vi "Home one linear axis relative to limit.vi"(6 "Set Home limit":bool caption="Set Home relative to this limit", 8 "error in (no error)":errorcluster, 9 "Axis (1..4)":u16(ring)=1 items=["X"=1, "Y"=2, "Z"=3, "Rotary"=4], 10 "Absolute 0 position, counts":i32=-200 caption="Absolute 0 position from limit switch, counts", 11 "VISA resource name":refnum<visa-resource-name>) -> (0 "error out":errorcluster, 1 "current position, counts":i32, 3 "VISA resource out":refnum<visa-resource-name>)   [LabVIEW 2017]
panel:
  # "< always positive number here"
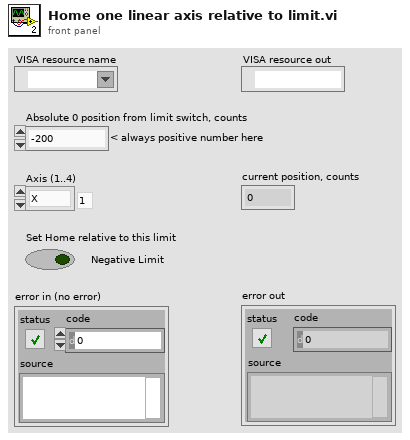
[diagram p1: front panel]
types:
  T1 = enum16{"Cmd-Response", "Write Only", "Read Only"}
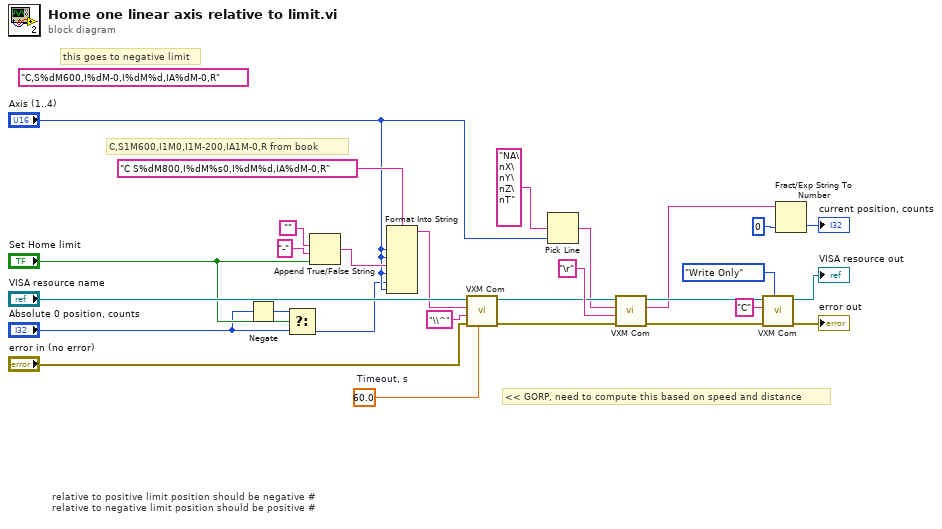
[diagram p0: block diagram]
diagram:
  (unwired) "C,S%dM600,I%dM-0,I%dM%d,IA%dM-0,R" ("Write Buffer")
  w11 = 60.0  # Timeout, s
  # "relative to positive limit position should be negative #\nrelative to negative limit position should be positive #"
  # "C,S1M600,I1M0,I1M-200,IA1M-0,R from book"
  # "this goes to negative limit"
  # "<< GORP, need to compute this based on speed and distance"
  n1 = Negate(x="Absolute 0 position, counts") -> (-x=w1:i32)
  n2 = Select(t=w1, s="Set Home limit", f="Absolute 0 position, counts") -> (s? t:f=w4:i32)
  n3 = Append True/False String(1:"Set Home limit", 2:"-" ("false string"), 3:"") -> (0:w6:string)  [unwired: 1 in]
  n4 = Format Into String(format string="C S%dM800,I%dM%s0,I%dM%d,IA%dM-0,R" ("Write Buffer"), "Axis (1..4)", "Axis (1..4)", w6, "Axis (1..4)", w4, "Axis (1..4)") -> (resulting string=w27:string)  [unwired: 2 in, 1 out]
  n5 = call "VXM Com.vi"("Timeout, s"=w11, "error in (no error)"="error in (no error)", "Termination String ('/' codes)"="\\^", "Write Buffer ('/' codes)"=w27, "VISA resource name"="VISA resource name") -> ("error out"=w19:errorcluster, "VISA resource out"=w23:refnum<visa-resource-name>)  [unwired: 4 in, 1 out]
  n6 = Pick Line(multi-line string="NA\nX\nY\nZ\nT", line index="Axis (1..4)") -> (output string=w13:string)  [unwired: 1 in]
  n7 = call "VXM Com.vi"("error in (no error)"=w19, "Termination String ('/' codes)"="\r", "Write Buffer ('/' codes)"=w13, "VISA resource name"=w23) -> ("error out"=w22:errorcluster, "Response String ('/' codes)"=w17:string, "VISA resource out"=w21:refnum<visa-resource-name>)  [unwired: 5 in]
  n8 = call "VXM Com.vi"("Operation"=T1."Write Only", "error in (no error)"=w22, "Write Buffer ('/' codes)"="C" ("Write Buffer"), "VISA resource name"=w21) -> ("error out"=→"error out":errorcluster, "VISA resource out"=→"VISA resource out":refnum<visa-resource-name>)  [unwired: 5 in, 1 out]
  n9 = Fract/Exp String To Number(string=w17, default (0 dbl)=0 ("default (0 DBL)")) -> (number=→"current position, counts":i32)  [unwired: 2 in, 1 out]
